vi "Extract 3x3 Grid from View.vi"(10 "Team Index":i32, 11 "View":i32[](array[numeric]) caption="View (Team Index, -1: empty)") -> (3 "I32 3x3 Grid 2":T1)   [LabVIEW 2017, in "AntFarm_MB.lvclass"]
uses:
  AntFarm_MB.lvclass
  TypeDefs/Cluster_I32 3x3 Grid.ctl
panel:
  # "NW\nN\nNE\nE\nSE\nS\nSW\nW"
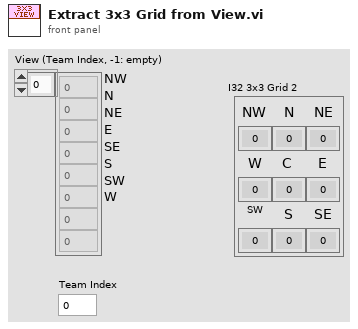
[diagram p1: front panel]
types:
  T1 = typedef "Cluster_I32 3x3 Grid.ctl" = cluster{"NW":i32, "N":i32, "NE":i32, "E":i32, "SE":i32, "S":i32, "SW":i32, "W":i32, "C":i32}
  T2 = cluster{"[0]":i32, "[1]":i32, "[2]":i32, "[3]":i32, "[4]":i32, "[5]":i32, "[6]":i32, "[7]":i32, "[8]":i32}
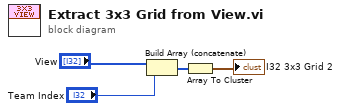
[diagram p0: block diagram]
diagram:
  n1 = Build Array (concatenate)("View", "Team Index") -> (w2:i32[])
  n2 = Array To Cluster(array=w2) -> (cluster=→"I32 3x3 Grid 2":T2)
